vi "DecrementInventory.vi"(8 "error in":errorcluster, 9 "Language":T1, 10 "Name":string, 11 "DB Path":path) -> (0 "error out":errorcluster)   [LabVIEW 2020]
uses:
  Controls/Language Enum.ctl
  <vilib>/drjdpowell/SQLite Library/SQL Connection/Open (path).vi
  <vilib>/drjdpowell/SQLite Library/SQL Connection/Open (string).vi
  <vilib>/AdvancedString/Path To Command Line String.vi
  <vilib>/drjdpowell/SQLite Library/SQL Connection/Execute SQL (Single Integer).vi
  <vilib>/drjdpowell/SQLite Library/SQL Connection/Execute SQL (Single DBL).vi
  <vilib>/drjdpowell/SQLite Library/SQL Connection/Connection.lvclass
  <vilib>/drjdpowell/SQLite Library/SQLite.lvlib
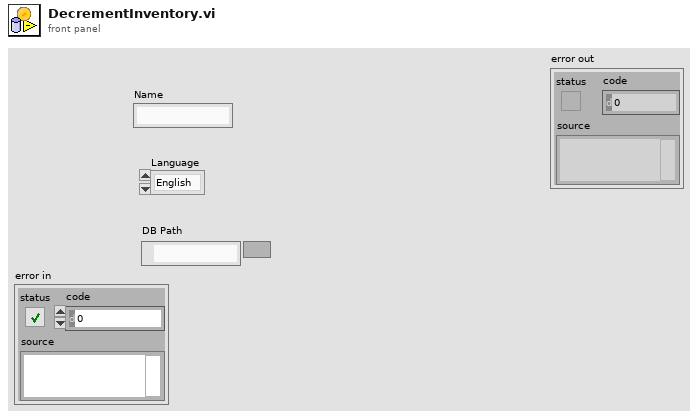
[diagram p1: front panel]
types:
  T1 = typedef "Language Enum.ctl" = enum16{"English", "Español", "Français"}
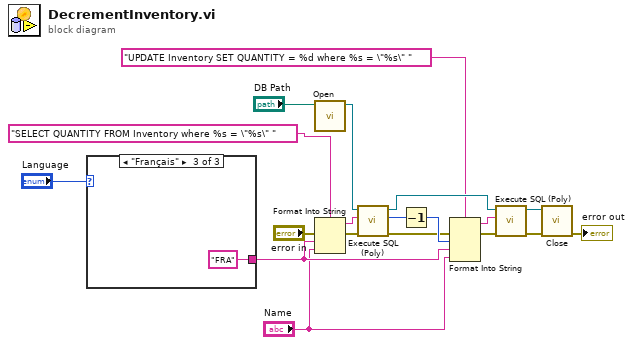
[diagram p0: block diagram]
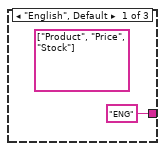
[diagram p2: hidden frame]
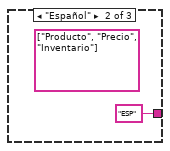
[diagram p3: hidden frame]
diagram:
  n1 = case shown="\"Français\"" "Language" {
    tunnel: ["ENG" "ESP" "FRA"] -> w9
    frame "English", Default {
      (unwired) string[] ["Product", "Price", "Stock"] ("Column Header Strings[]")
    }
    frame "Español" {
      (unwired) string[] ["Producto", "Precio", "Inventario"] ("Column Header Strings[]")
    }
    frame "Français" {
    }
  }
  n2 = call-poly <vilib>:"Open.vi"("db file"="DB Path") -> ("SQLite Connection"=w17:refnum<class "Connection.lvclass">)  [unwired: 9 in, 1 out]
  n3 = Format Into String(format string="SELECT QUANTITY FROM Inventory where %s = \"%s\" ", error in="error in", w9, "Name") -> (resulting string=w16:string, error out=w15:errorcluster)  [unwired: 1 in]
  n4 = call-poly <vilib>:"Execute SQL (Poly).vi"("error in (no error)"=w15, "SQL"=w16, "SQLite Connection in"=w17) -> ("error out"=w3:errorcluster, "Result"=w12:i64, "SQLite Connection"=w13:refnum<class "Connection.lvclass">)  [unwired: 6 in]
  n5 = Decrement(x=w12) -> (x-1=w10:i64)
  n6 = Format Into String(format string="UPDATE Inventory SET QUANTITY = %d where %s = \"%s\" ", error in=w3, w10, w9, "Name") -> (resulting string=w7:string, error out=w4:errorcluster)  [unwired: 1 in]
  n7 = call-poly <vilib>:"Execute SQL (Poly).vi"("error in (no error)"=w4, "SQL"=w7, "SQLite Connection in"=w13) -> ("error out"=w5:errorcluster, "SQLite Connection"=w6:refnum<class "Connection.lvclass">)  [unwired: 6 in, 1 out]
  n8 = call-dynamic "Close.vi"("error in (no error)"=w5, "SQLite Connection in"=w6) -> ("error out"=→"error out":errorcluster)  [unwired: 9 in]
